vi "ENUM_To String.vi"(4 "ENUM":variant) -> (1 "String Out":string)   [LabVIEW 2015]
doc: "Converts enum to string"
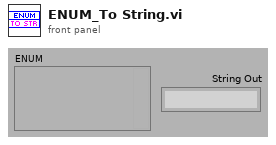
[diagram p1: front panel]
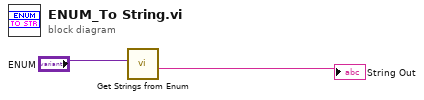
[diagram p0: block diagram]
diagram:
  n1 = call "Get Strings from Enum.vi"("Enum"="ENUM") -> ("String Value"=→"String Out":string)  [unwired: 7 in, 3 out]
